vi "Delete row zeroes (SubVI).vi"(11 "direct_shot_array":dbl[][](array[numeric])) -> (3 "Array":dbl[][](array[numeric]))   [LabVIEW 2013]
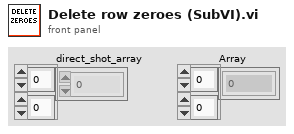
[diagram p1: front panel]
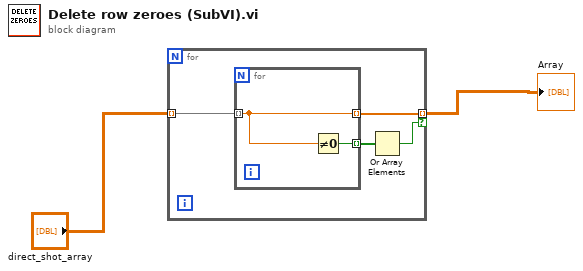
[diagram p0: block diagram]
diagram:
  n1 = for {
    tunnel: "direct_shot_array" -> [w6] mode=indexing
    tunnel: [w4] -> w1 mode=indexing if=w3
    n2 = for {
      tunnel: w6 -> [w7] mode=indexing
      tunnel: [w8] -> w5 mode=indexing
      tunnel: [w7] -> w4 mode=indexing
      n3 = Not Equal To 0?(x=w7) -> (x != 0?=w8:bool)
    }
    n4 = Or Array Elements(Boolean array=w5) -> (logical OR=w3:bool)
  }
  "Array" <- w1
